vi "update_position.vi"(8 "error in (no error)":errorcluster, 11 "YK090817SutterMP285Stage in":refnum<class "YK090817SutterMP285Stage.lvclass">=refnum) -> (0 "error out":errorcluster, 3 "YK090817SutterMP285Stage out":refnum<class "YK090817SutterMP285Stage.lvclass">)   [LabVIEW 2010, in "YK090817SutterMP285Stage.lvclass"]
uses:
  YK090817SutterMP285Stage.lvclass
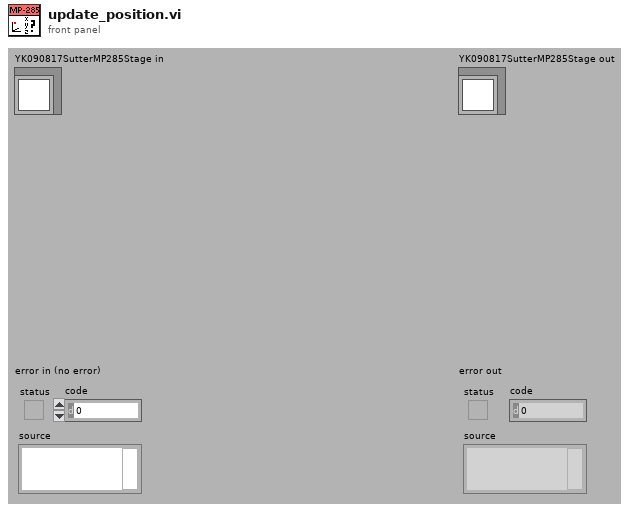
[diagram p1: front panel]
types:
  T1 = cluster{"[0]":dbl[unit], "[1]":dbl[unit], "[2]":dbl[unit]}
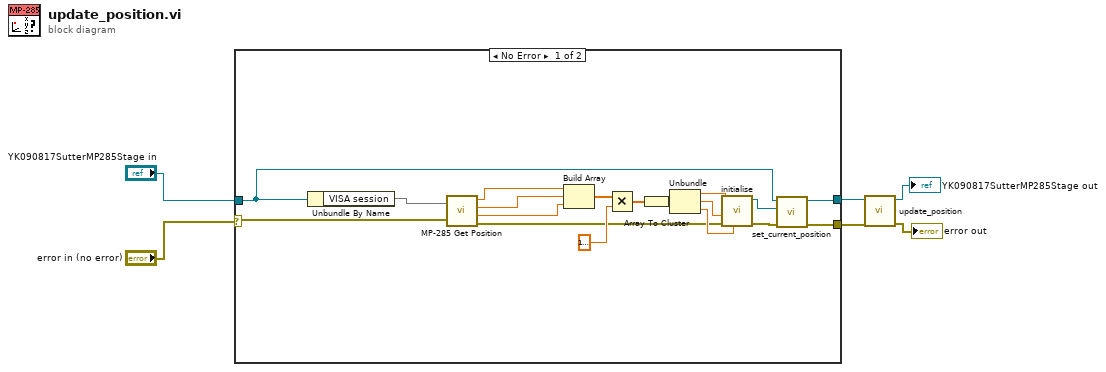
[diagram p0: block diagram]
diagram:
  n1 = case shown="No Error" "error in (no error)" {
    selector: "error in (no error)" -> [w14 w26]
    tunnel: [w23 w26] -> w4
    tunnel: [w9 w25] -> w3
    tunnel: "YK090817SutterMP285Stage in" -> [w8 w25]
    frame No Error {
      n2 = Unbundle By Name(w8) -> ("VISA session"=w7)
      n3 = call "MP-285 Get Position.vi"("error in (no error)"=w14, "VISA resource name"=w7) -> ("error out"=w13:errorcluster, "Output: Z axis (microns)"=w12:dbl, "Output: Y axis (microns)"=w11:dbl, "Output: X axis (microns)"=w10:dbl)  [unwired: 1 out]
      n4 = Build Array(w10, w11, w12) -> (w17:dbl[])
      n5 = Multiply(x=w17, y=dbl[unit] 1e-06 ("decoded data")) -> (x*y=w16:dbl[unit][])
      n6 = Array To Cluster(array=w16) -> (cluster=w21:T1)
      n7 = Unbundle(w21) -> ("[0]"=w20:dbl[unit], "[1]"=w18:dbl[unit], "[2]"=w19:dbl[unit])
      n8 = call "initialise.vi"("z"=w19, "error in (no error)"=w13, "y"=w18, "x"=w20) -> ("error out"=w24:errorcluster, "SpaceVector out"=w22:refnum<class "SpaceVector.lvclass">)  [unwired: 6 out]
      n9 = call-dynamic "set_current_position.vi"("error in (no error)"=w24, "SpaceVector.lvclass"=w22, "DL090409StageScaffold.lvclass in"=w8) -> ("error out"=w23:errorcluster, "DL090409StageScaffold.lvclass out"=w9:refnum<class "YK090817SutterMP285Stage.lvclass">)  [unwired: 7 out]
    }
    frame Error {
    }
  }
  n10 = call-parent "update_position.vi"("error in (no error)"=w4, "DL090409StageScaffold in"=w3) -> ("error out"=→"error out":errorcluster, "DL090409StageScaffold out"=→"YK090817SutterMP285Stage out":refnum<class "YK090817SutterMP285Stage.lvclass">)  [unwired: 8 out]
